vi "SetEnable.vi"(11 "Enabled/Disable":bool) -> ()   [LabVIEW 2011]
uses:
  GlobalVariables.vi
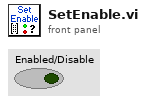
[diagram p1: front panel]
types:
  T1 = typedef "Device Cluster.ctl" = cluster{"Dnet":string, "Node":i32, "Type":string, "ID Number":u8, "SCCM":dbl, "FullScale":dbl, "Input Bytes":i32, "Output Bytes":i32, "Input Start Location":i32, "Output Start Location":i32, "Enabled":bool, "Bytes":u8[]}
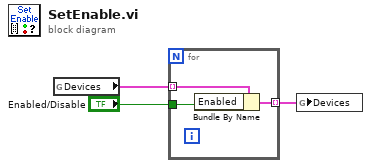
[diagram p0: block diagram]
diagram:
  n1 = global read "GlobalVariables.vi" "Devices"() -> (w3:T1[])
  n2 = for {
    tunnel: w3 -> [w4] mode=indexing
    tunnel: "Enabled/Disable" -> [w6]
    tunnel: [w5] -> w1 mode=indexing
    n3 = Bundle By Name(cluster=w4, "Enabled"=w6) -> (w5:T1)
  }
  n4 = global write "GlobalVariables.vi" "Devices"(w1) -> ()
